vi "PID Structure Conversion (DBL).vi"(4 "derivative unit":T2 items=["min", "s"], 5 "proportional unit":T4 items=["Gain (K)", "Band (PB)"], 6 "integral unit":T2 items=["min", "s"], 7 "PID structure":T3 items=["Academic (Standard)", "Parallel", "Series"], 9 "derivative":dbl, 10 "integral":dbl, 11 "proportional":dbl) -> (3 "PID gains":T1)   [LabVIEW 2020, in "NI_PID_pid.lvlib"]
doc: "Converts a PID controller or controllers in Academic, Parallel, or Series form into the form (Academic) and <B>PID gains</B> units that the PID VIs expect. Wire data to the <B>proportional</B>, <B>integral</B>, or <B>derivative</B> input to determine the polymorphic instance to use, or manually select the instance."
uses:
  NI_PID_pid.lvlib
  PID Gain Unit.ctl
  PID Structure.ctl
  PID Time Unit.ctl
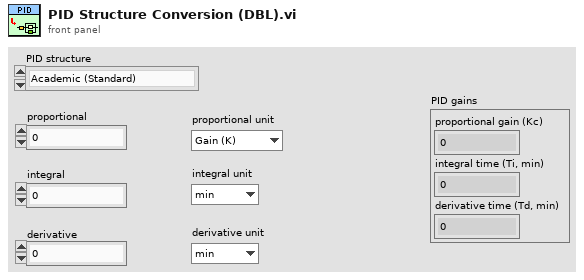
[diagram p1: front panel]
types:
  T1 = cluster{"proportional gain (Kc)":dbl, "integral time (Ti, min)":dbl, "derivative time (Td, min)":dbl}
  T2 = typedef "NI_PID_pid.lvlib/PID Time Unit.ctl" = u16
  T3 = typedef "NI_PID_pid.lvlib/PID Structure.ctl" = u16
  T4 = typedef "NI_PID_pid.lvlib/PID Gain Unit.ctl" = u16
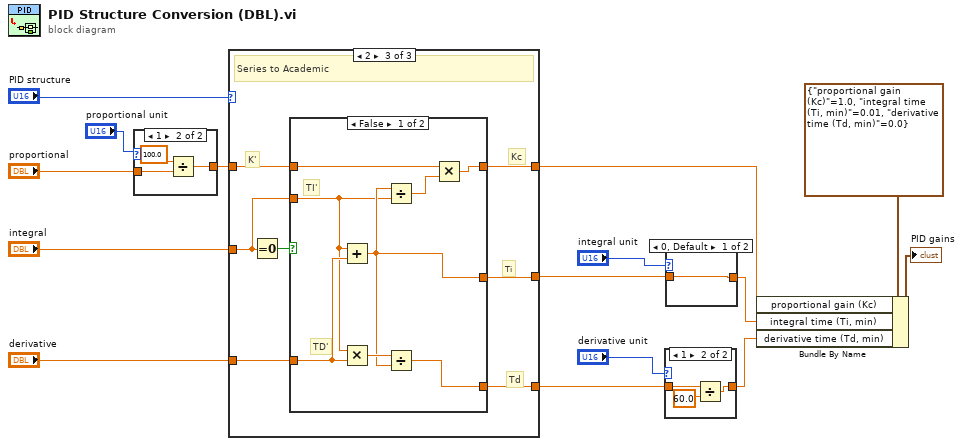
[diagram p0: block diagram]
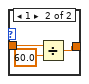
[diagram p4: hidden frame]
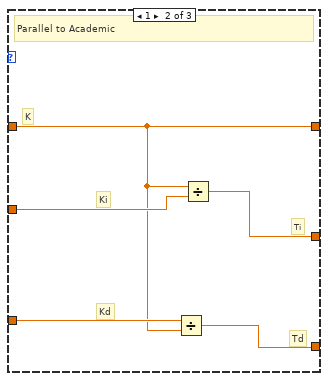
[diagram p6: hidden frame]
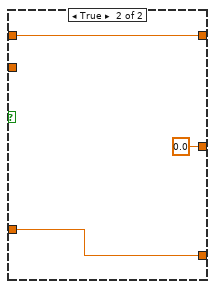
[diagram p7: hidden frame]
diagram:
  n1 = case shown="1" "proportional unit" {
    tunnel: "proportional" -> [w16 w17]
    tunnel: [w16 w19] -> w2
    frame 0, Default {
    }
    frame 1 {
      n2 = Divide(x=100.0, y=w17) -> (x/y=w19:dbl)
    }
  }
  n3 = case shown="2" "PID structure" {
    tunnel: "derivative" -> [w22 w25 w32]
    tunnel: "integral" -> [w21 w27 w28]
    tunnel: [w22 w23 w30] -> w6
    tunnel: [w21 w26 w31] -> w5
    tunnel: [w20 w24 w33] -> w1
    tunnel: w2 -> [w20 w24 w34]
    frame 0, Default {
      # "Td"
      # "Ti"
      # "Kc"
    }
    frame 1 {
      # "Td"
      # "Ti"
      # "Kd"
      # "Ki"
      # "K"
      # "Parallel to Academic"
      n4 = Divide(x=w25, y=w24) -> (x/y=w23:dbl)
      n5 = Divide(x=w24, y=w27) -> (x/y=w26:dbl)
    }
    frame 2 {
      # "K'"
      # "Td"
      # "Kc"
      # "Ti"
      # "Series to Academic"
      n6 = Equal To 0?(x=w28) -> (x = 0?=w29:bool)
      n7 = case shown="False" w29 {
        tunnel: w34 -> [w42 w45]
        tunnel: [w40 w45] -> w33
        tunnel: w32 -> [w39 w43]
        tunnel: [w37 0.0] -> w31
        tunnel: [w36 w43] -> w30
        tunnel: w28 -> [w35 _]
        frame False {
          # "TD'"
          # "TI'"
          n8 = Add(x=w35, y=w39) -> (x+y=w37:dbl)
          n9 = Multiply(x=w35, y=w39) -> (x*y=w38:dbl)
          n10 = Divide(x=w37, y=w35) -> (x/y=w41:dbl)
          n11 = Divide(x=w38, y=w37) -> (x/y=w36:dbl)
          n12 = Multiply(x=w42, y=w41) -> (x*y=w40:dbl)
        }
        frame True {
        }
      }
    }
  }
  n13 = case shown="1" "derivative unit" {
    tunnel: w6 -> [w46 w49]
    tunnel: [w46 w47] -> w7
    frame 0, Default {
    }
    frame 1 {
      n14 = Divide(x=w49, y=60.0) -> (x/y=w47:dbl)
    }
  }
  n15 = case shown="0, Default" "integral unit" {
    tunnel: w5 -> [w50 w53]
    tunnel: [w50 w51] -> w8
    frame 0, Default {
    }
    frame 1 {
      n16 = Divide(x=w53, y=60.0) -> (x/y=w51:dbl)
    }
  }
  n17 = Bundle By Name(cluster=T1 {"proportional gain (Kc)"=1.0, "integral time (Ti, min)"=0.01, "derivative time (Td, min)"=0.0} ("PID gains"), "proportional gain (Kc)"=w1, "integral time (Ti, min)"=w8, "derivative time (Td, min)"=w7) -> (→"PID gains":T1)
